vi "pwm divider calculator.vi"(7 "PWM frequence":dbl) -> (0 "enable divider":bool, 1 "period":i32, 2 "divider rate":i32)   [LabVIEW 2019, in "my FPGA lib.lvlib" / "motor.lvclass"]
uses:
  motor.lvclass
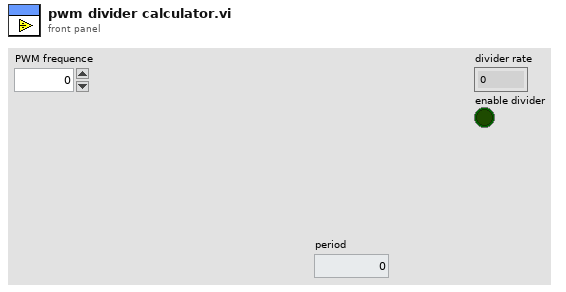
[diagram p1: front panel]
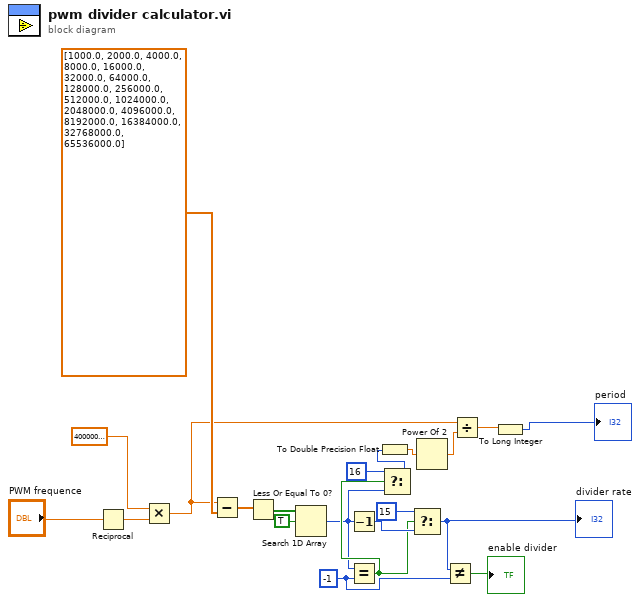
[diagram p0: block diagram]
diagram:
  w12 = -1 ("y")
  n1 = Reciprocal(x="PWM frequence") -> (1/x=w20:dbl)
  n2 = Multiply(x=40000000.0, y=w20) -> (x*y=w10:dbl)
  n3 = Subtract(x=w10, y=dbl[] [1000.0, 2000.0, 4000.0, 8000.0, 16000.0, 32000.0, 64000.0, 128000.0, 256000.0, 512000.0, 1024000.0, 2048000.0, 4096000.0, 8192000.0, 16384000.0, 32768000.0, 65536000.0]) -> (x-y=w17:dbl[])
  n4 = Less Or Equal To 0?(x=w17) -> (x <= 0?=w16:bool[])
  n5 = Search 1D Array(1D array=w16, element=TRUE) -> (index of element=w7:i32)  [unwired: 1 in]
  n6 = Decrement(x=w7) -> (x-1=w14:i32)
  n7 = Equal?(x=w7, y=w12) -> (x = y?=w9:bool)
  n8 = Select(t=16, s=w9, f=w7) -> (s? t:f=w5:i32)
  n9 = To Double Precision Float(number=w5) -> (double precision float=w4:dbl)
  n10 = Select(t=15, s=w9, f=w14) -> (s? t:f=w13:i32)
  "divider rate" <- w13
  n11 = Power Of 2(x=w4) -> (2^x=w3:dbl)
  n12 = Not Equal?(x=w13, y=w12) -> (x != y?=→"enable divider":bool)
  n13 = Divide(x=w10, y=w3) -> (x/y=w2:dbl)
  n14 = To Long Integer(number=w2) -> (32bit integer=→"period":i32)
